vi "append_to_log.vi"(5 "data_type":T1, 7 "dims":T2, 8 "error in (no error)":errorcluster, 9 "Location":string, 10 "Data":variant, 11 "lfield_logger in":refnum<class "lfield_logger.lvclass">) -> (0 "error out":errorcluster, 3 "lfield_logger out":refnum<class "lfield_logger.lvclass">)   [LabVIEW 2015, in "lfield_logger.lvclass"]
uses:
  lfield_logger.lvclass
  Data Logger Class/data_dimensionality.ctl
  Data Logger Class/logger_data_types.ctl
  Data Logger Class/data_logger.lvclass
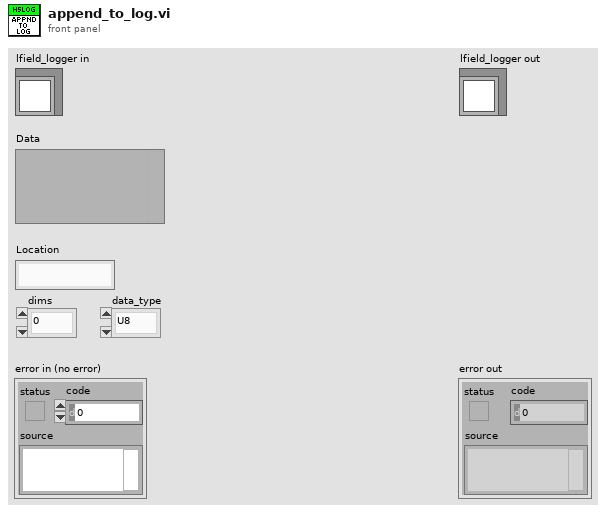
[diagram p1: front panel]
types:
  T1 = typedef "logger_data_types.ctl" = enum16{"U8", "I8", "U16", "I16", "U32", "I32", "DBL", "String"}
  T2 = typedef "data_dimensionality.ctl" = enum16{"0", "1", "2"}
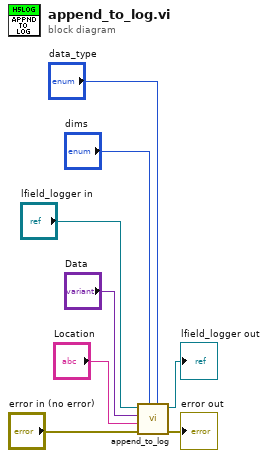
[diagram p0: block diagram]
diagram:
  n1 = call-parent "append_to_log.vi"("data_type"="data_type", "dims"="dims", "error in (no error)"="error in (no error)", "Location"="Location", "Data"="Data", "data_logger in"="lfield_logger in") -> ("error out"=→"error out":errorcluster, "data_logger out"=→"lfield_logger out":refnum<class "lfield_logger.lvclass">)  [unwired: 4 in]
